vi "Parking Go.vi"(8 "error in (no error)":errorcluster, 11 "Motion in":refnum<class "Motion.lvclass">) -> (0 "error out":errorcluster, 3 "Motion out":refnum<class "Motion.lvclass">)   [LabVIEW 2016, in "Motion.lvclass"]
uses:
  Motion.lvclass
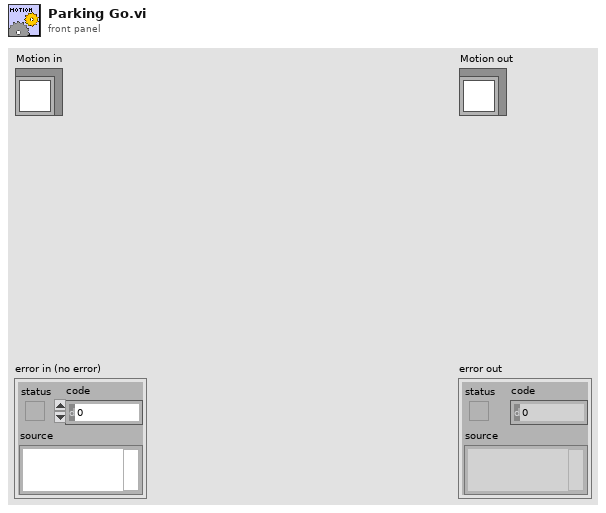
[diagram p1: front panel]
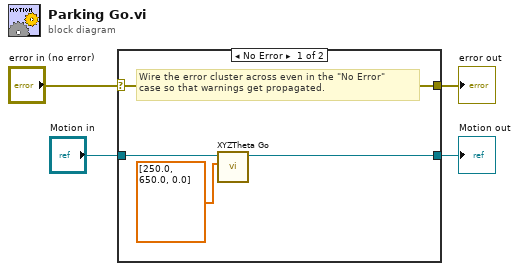
[diagram p0: block diagram]
diagram:
  n1 = case shown="No Error" "error in (no error)" {
    selector: "error in (no error)" -> [w8 w10]
    tunnel: [w8 w10] -> w3
    tunnel: [w6 w9] -> w1
    tunnel: "Motion in" -> [w7 w9]
    frame No Error {
      # "Wire the error cluster across even in the \"No Error\"\ncase so that warnings get propagated."
      n2 = call "XYZTheta Go.vi"("XYZTheta In"=dbl[] [250.0, 650.0, 0.0], "Motion in"=w7) -> ("Motion out"=w6:refnum<class "Motion.lvclass">)  [unwired: 7 in, 2 out]
    }
    frame Error {
    }
  }
  "error out" <- w3
  "Motion out" <- w1
